vi "Workbench.vi"   [LabVIEW 2024]
uses:
  SDL3/Video/WindowFlags--ring.ctl
  SDL3/Pixels/PixelFormat--enum.ctl
  SDL3/Render/TextureAccess-enum.ctl
  SDL3/Init/InitFlags--ring.ctl
  SDL3/Events/MouseMotionEvent--cluster.ctl
  SDL3/Video/WindowID--integer.ctl
  SDL3/Mouse/MouseID--integer.ctl
  SDL3/Mouse/MouseButtonFlags--ring.ctl
  SDL3/Video/GLAttr--enum.ctl
  SDL3/Render/Vertex--cluster.ctl
  SDL3/Rect/FPoint--cluster.ctl
  SDL3/Pixels/FColor--cluster.ctl
  SDL3/Error/GetError-UiThread.vi
  SDL3/Pixels/PixelFormatEnumToU32.vi
  <vilib>/Utility/error.llb/Error Cluster From Error Code.vi
  SDL3/Init/Init.lvlib
  SDL3/Video/Video.lvlib
  SDL3/Render/Render.lvlib
  SDL3/Pixels/Pixels.lvlib
  SDL3/Timer/Timer.lvlib
  SDL3/Events/Events.lvlib
  SDL3/Mouse/Mouse.lvlib
  SDL3/Rect/Rect.lvlib
  SDL3/Hints/Hints.lvlib
types:
  T1 = typedef "SDL3.lvlib/Video.lvlib/GLAttr--enum.ctl" = enum32{"SDL_GL_RED_SIZE", "SDL_GL_GREEN_SIZE", "SDL_GL_BLUE_SIZE", "SDL_GL_ALPHA_SIZE", "SDL_GL_BUFFER_SIZE", "SDL_GL_DOUBLEBUFFER", "SDL_GL_DEPTH_SIZE", "SDL_GL_STENCIL_SIZE", "SDL_GL_ACCUM_RED_SIZE", "SDL_GL_ACCUM_GREEN_SIZE", "SDL_GL_ACCUM_BLUE_SIZE", "SDL_GL_ACCUM_ALPHA_SIZE", "SDL_GL_STEREO", "SDL_GL_MULTISAMPLEBUFFERS", "SDL_GL_MULTISAMPLESAMPLES", "SDL_GL_ACCELERATED_VISUAL", "SDL_GL_RETAINED_BACKING", "SDL_GL_CONTEXT_MAJOR_VERSION", "SDL_GL_CONTEXT_MINOR_VERSION", "SDL_GL_CONTEXT_FLAGS", "SDL_GL_CONTEXT_PROFILE_MASK", "SDL_GL_SHARE_WITH_CURRENT_CONTEXT", "SDL_GL_FRAMEBUFFER_SRGB_CAPABLE", "SDL_GL_CONTEXT_RELEASE_BEHAVIOR", "SDL_GL_CONTEXT_RESET_NOTIFICATION", "SDL_GL_CONTEXT_NO_ERROR", "SDL_GL_FLOATBUFFERS", "SDL_GL_EGL_PLATFORM"}
  T2 = enum32{"Invalid", "Standard", "Closed", "Hidden", "Minimized", "Maximized"}
  T3 = typedef "SDL3.lvlib/Events.lvlib/MouseMotionEvent--cluster.ctl" = cluster{"timestamp":u64, "windowID":T4, "which":T5, "state":T6, "x":sgl, "y":sgl, "xrel":sgl, "yrel":sgl}
  T4 = typedef "SDL3.lvlib/Video.lvlib/WindowID--integer.ctl" = u32
  T5 = typedef "SDL3.lvlib/Mouse.lvlib/MouseID--integer.ctl" = u32
  T6 = typedef "SDL3.lvlib/Mouse.lvlib/MouseButtonFlags--ring.ctl" = u32
  T7 = typedef "SDL3.lvlib/Init.lvlib/InitFlags--ring.ctl" = u32
  T8 = typedef "SDL3.lvlib/Render.lvlib/TextureAccess-enum.ctl" = enum32{"SDL_TEXTUREACCESS_STATIC", "SDL_TEXTUREACCESS_STREAMING", "SDL_TEXTUREACCESS_TARGET"}
  T9 = typedef "SDL3.lvlib/Pixels.lvlib/PixelFormat--enum.ctl" = enum32{"SDL_PIXELFORMAT_UNKNOWN", "SDL_PIXELFORMAT_INDEX1LSB", "SDL_PIXELFORMAT_INDEX1MSB", "SDL_PIXELFORMAT_INDEX2LSB", "SDL_PIXELFORMAT_INDEX2MSB", "SDL_PIXELFORMAT_INDEX4LSB", "SDL_PIXELFORMAT_INDEX4MSB", "SDL_PIXELFORMAT_INDEX8", "SDL_PIXELFORMAT_RGB332", "SDL_PIXELFORMAT_XRGB4444", "SDL_PIXELFORMAT_XBGR4444", "SDL_PIXELFORMAT_XRGB1555", "SDL_PIXELFORMAT_XBGR1555", "SDL_PIXELFORMAT_ARGB4444", "SDL_PIXELFORMAT_RGBA4444", "SDL_PIXELFORMAT_ABGR4444", "SDL_PIXELFORMAT_BGRA4444", "SDL_PIXELFORMAT_ARGB1555", "SDL_PIXELFORMAT_RGBA5551", "SDL_PIXELFORMAT_ABGR1555", "SDL_PIXELFORMAT_BGRA5551", "SDL_PIXELFORMAT_RGB565", "SDL_PIXELFORMAT_BGR565", "SDL_PIXELFORMAT_RGB24", "SDL_PIXELFORMAT_BGR24", "SDL_PIXELFORMAT_XRGB8888", "SDL_PIXELFORMAT_RGBX8888", "SDL_PIXELFORMAT_XBGR8888", "SDL_PIXELFORMAT_BGRX8888", "SDL_PIXELFORMAT_ARGB8888", "SDL_PIXELFORMAT_RGBA8888", "SDL_PIXELFORMAT_ABGR8888", "SDL_PIXELFORMAT_BGRA8888", "SDL_PIXELFORMAT_XRGB2101010", "SDL_PIXELFORMAT_XBGR2101010", "SDL_PIXELFORMAT_ARGB2101010", "SDL_PIXELFORMAT_ABGR2101010", "SDL_PIXELFORMAT_RGB48", "SDL_PIXELFORMAT_BGR48", "SDL_PIXELFORMAT_RGBA64", "SDL_PIXELFORMAT_ARGB64", "SDL_PIXELFORMAT_BGRA64", "SDL_PIXELFORMAT_ABGR64", "SDL_PIXELFORMAT_RGB48_FLOAT", "SDL_PIXELFORMAT_BGR48_FLOAT", "SDL_PIXELFORMAT_RGBA64_FLOAT", "SDL_PIXELFORMAT_ARGB64_FLOAT", "SDL_PIXELFORMAT_BGRA64_FLOAT", "SDL_PIXELFORMAT_ABGR64_FLOAT", "SDL_PIXELFORMAT_RGB96_FLOAT", "SDL_PIXELFORMAT_BGR96_FLOAT", "SDL_PIXELFORMAT_RGBA128_FLOAT", "SDL_PIXELFORMAT_ARGB128_FLOAT", "SDL_PIXELFORMAT_BGRA128_FLOAT", "SDL_PIXELFORMAT_ABGR128_FLOAT", "SDL_PIXELFORMAT_YV12", "SDL_PIXELFORMAT_IYUV", "SDL_PIXELFORMAT_YUY2", "SDL_PIXELFORMAT_UYVY", "SDL_PIXELFORMAT_YVYU", "SDL_PIXELFORMAT_NV12", "SDL_PIXELFORMAT_NV21", "SDL_PIXELFORMAT_P010", "SDL_PIXELFORMAT_EXTERNAL_OES"}
  T10 = typedef "SDL3.lvlib/Video.lvlib/WindowFlags--ring.ctl" = u64
  T11 = typedef "SDL3.lvlib/Render.lvlib/Vertex--cluster.ctl" = cluster{"Position":T12, "Color":T13, "TexCoord":T12}
  T12 = typedef "SDL3.lvlib/Rect.lvlib/FPoint--cluster.ctl" = cluster{"x":sgl, "y":sgl}
  T13 = typedef "SDL3.lvlib/Pixels.lvlib/FColor--cluster.ctl" = cluster{"r":sgl, "g":sgl, "b":sgl, "a":sgl}
  T14 = typedef "SDL3.lvlib/Events.lvlib/EventType--enum.ctl" = enum16{"LV_NONE", "LV_UNSUPPORTED", "SDL_EVENT_QUIT", "SDL_EVENT_LOCALE_CHANGED", "SDL_EVENT_SYSTEM_THEME_CHANGED", "SDL_EVENT_DISPLAY_ORIENTATION", "SDL_EVENT_DISPLAY_ADDED", "SDL_EVENT_DISPLAY_REMOVED", "SDL_EVENT_DISPLAY_MOVED", "SDL_EVENT_DISPLAY_DESKTOP_MODE_CHANGED", "SDL_EVENT_DISPLAY_CURRENT_MODE_CHANGED", "SDL_EVENT_DISPLAY_CONTENT_SCALE_CHANGED", "SDL_EVENT_WINDOW_SHOWN", "SDL_EVENT_WINDOW_HIDDEN", "SDL_EVENT_WINDOW_EXPOSED", "SDL_EVENT_WINDOW_MOVED", "SDL_EVENT_WINDOW_RESIZED", "SDL_EVENT_WINDOW_PIXEL_SIZE_CHANGED", "SDL_EVENT_WINDOW_METAL_VIEW_RESIZED", "SDL_EVENT_WINDOW_MINIMIZED", "SDL_EVENT_WINDOW_MAXIMIZED", "SDL_EVENT_WINDOW_RESTORED", "SDL_EVENT_WINDOW_MOUSE_ENTER", "SDL_EVENT_WINDOW_MOUSE_LEAVE", "SDL_EVENT_WINDOW_FOCUS_GAINED", "SDL_EVENT_WINDOW_FOCUS_LOST", "SDL_EVENT_WINDOW_CLOSE_REQUESTED", "SDL_EVENT_WINDOW_HIT_TEST", "SDL_EVENT_WINDOW_ICCPROF_CHANGED", "SDL_EVENT_WINDOW_DISPLAY_CHANGED", "SDL_EVENT_WINDOW_DISPLAY_SCALE_CHANGED", "SDL_EVENT_WINDOW_SAFE_AREA_CHANGED", "SDL_EVENT_WINDOW_OCCLUDED", "SDL_EVENT_WINDOW_ENTER_FULLSCREEN", "SDL_EVENT_WINDOW_LEAVE_FULLSCREEN", "SDL_EVENT_WINDOW_DESTROYED", "SDL_EVENT_WINDOW_HDR_STATE_CHANGED", "SDL_EVENT_KEY_DOWN", "SDL_EVENT_KEY_UP", "SDL_EVENT_TEXT_EDITING", "SDL_EVENT_TEXT_INPUT", "SDL_EVENT_KEYMAP_CHANGED", "SDL_EVENT_KEYBOARD_ADDED", "SDL_EVENT_KEYBOARD_REMOVED", "SDL_EVENT_TEXT_EDITING_CANDIDATES", "SDL_EVENT_MOUSE_MOTION", "SDL_EVENT_MOUSE_BUTTON_DOWN", "SDL_EVENT_MOUSE_BUTTON_UP", "SDL_EVENT_MOUSE_WHEEL", "SDL_EVENT_MOUSE_ADDED", "SDL_EVENT_MOUSE_REMOVED", "SDL_EVENT_JOYSTICK_AXIS_MOTION", "SDL_EVENT_JOYSTICK_BALL_MOTION", "SDL_EVENT_JOYSTICK_HAT_MOTION", "SDL_EVENT_JOYSTICK_BUTTON_DOWN", "SDL_EVENT_JOYSTICK_BUTTON_UP", "SDL_EVENT_JOYSTICK_ADDED", "SDL_EVENT_JOYSTICK_REMOVED", "SDL_EVENT_JOYSTICK_BATTERY_UPDATED", "SDL_EVENT_JOYSTICK_UPDATE_COMPLETE", "SDL_EVENT_GAMEPAD_AXIS_MOTION", "SDL_EVENT_GAMEPAD_BUTTON_DOWN", "SDL_EVENT_GAMEPAD_BUTTON_UP", "SDL_EVENT_GAMEPAD_ADDED", "SDL_EVENT_GAMEPAD_REMOVED", "SDL_EVENT_GAMEPAD_REMAPPED", "SDL_EVENT_GAMEPAD_TOUCHPAD_DOWN", "SDL_EVENT_GAMEPAD_TOUCHPAD_MOTION", "SDL_EVENT_GAMEPAD_TOUCHPAD_UP", "SDL_EVENT_GAMEPAD_SENSOR_UPDATE", "SDL_EVENT_GAMEPAD_UPDATE_COMPLETE", "SDL_EVENT_GAMEPAD_STEAM_HANDLE_UPDATED", "SDL_EVENT_FINGER_DOWN", "SDL_EVENT_FINGER_UP", "SDL_EVENT_FINGER_MOTION", "SDL_EVENT_CLIPBOARD_UPDATE", "SDL_EVENT_DROP_FILE", "SDL_EVENT_DROP_TEXT", "SDL_EVENT_DROP_BEGIN", "SDL_EVENT_DROP_COMPLETE", "SDL_EVENT_DROP_POSITION", "SDL_EVENT_AUDIO_DEVICE_ADDED", "SDL_EVENT_AUDIO_DEVICE_REMOVED", "SDL_EVENT_AUDIO_DEVICE_FORMAT_CHANGED", "SDL_EVENT_SENSOR_UPDATE", "SDL_EVENT_PEN_PROXIMITY_IN", "SDL_EVENT_PEN_PROXIMITY_OUT", "SDL_EVENT_PEN_DOWN", "SDL_EVENT_PEN_UP", "SDL_EVENT_PEN_BUTTON_DOWN", "SDL_EVENT_PEN_BUTTON_UP", "SDL_EVENT_PEN_MOTION", "SDL_EVENT_PEN_AXIS", "SDL_EVENT_CAMERA_DEVICE_ADDED", "SDL_EVENT_CAMERA_DEVICE_REMOVED", "SDL_EVENT_CAMERA_DEVICE_APPROVED", "SDL_EVENT_CAMERA_DEVICE_DENIED", "SDL_EVENT_RENDER_TARGETS_RESET", "SDL_EVENT_RENDER_DEVICE_RESET", "SDL_EVENT_POLL_SENTINEL", "SDL_EVENT_USER"}
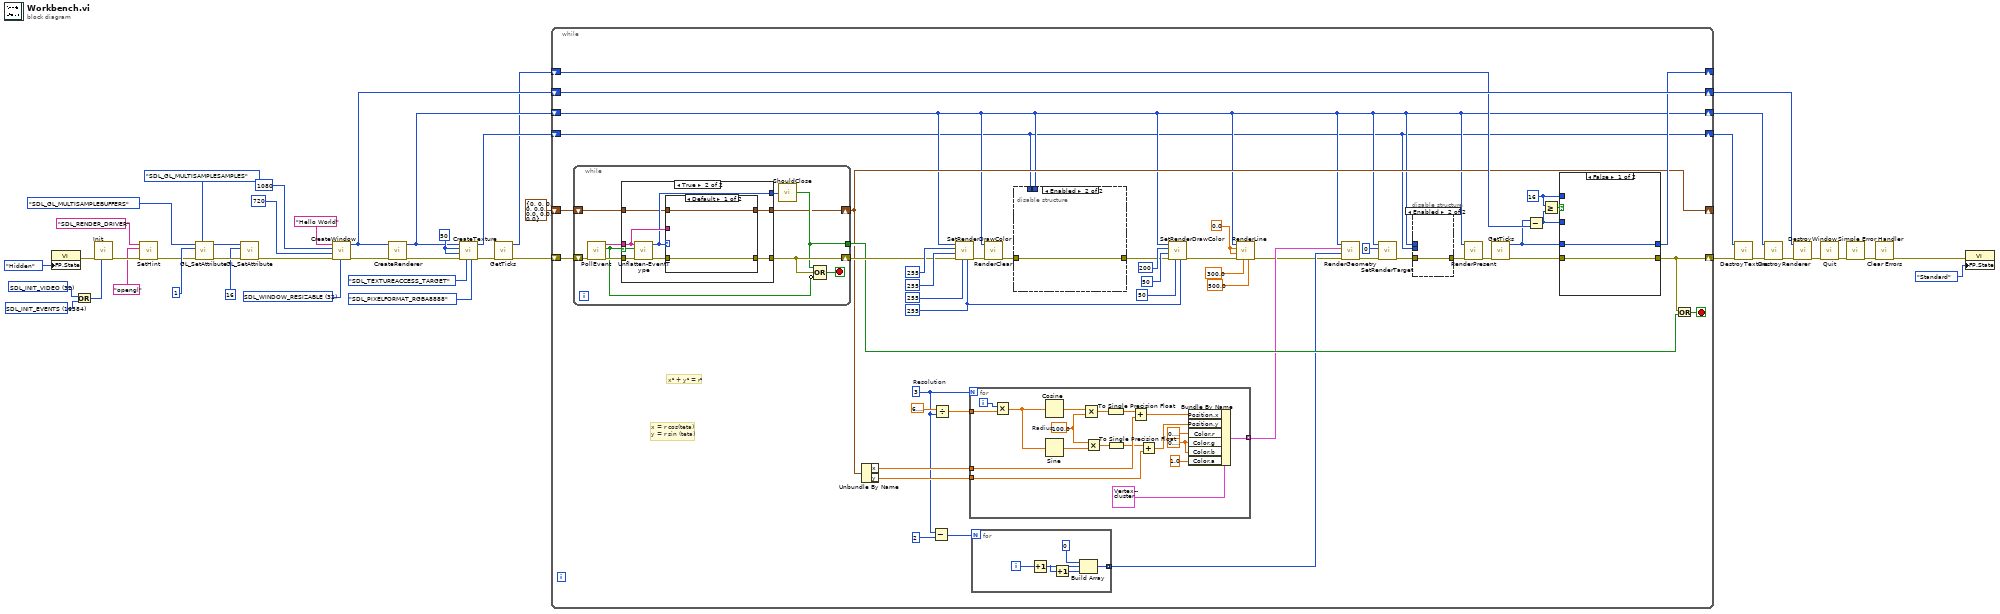
[diagram p0: block diagram]
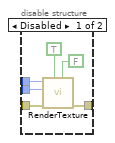
[diagram p2: hidden frame]
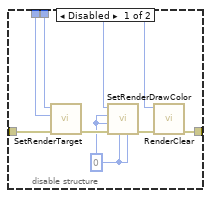
[diagram p3: hidden frame]
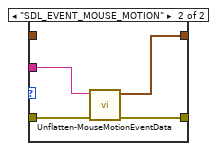
[diagram p5: hidden frame]
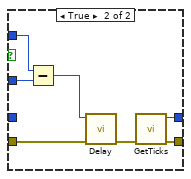
[diagram p6: hidden frame]
diagram:
  w13 = T7 16384 items=["NONE"=0, "SDL_INIT_AUDIO"=16, "SDL_INIT_VIDEO"=32, "SDL_INIT_JOYSTICK"=512, "SDL_INIT_HAPTIC"=4096, "SDL_INIT_GAMEPAD"=8192, "SDL_INIT_EVENTS"=16384, "SDL_INIT_SENSOR"=32768, "SDL_INIT_CAMER"=65536] ("y")
  w18 = T7 32 items=["NONE"=0, "SDL_INIT_AUDIO"=16, "SDL_INIT_VIDEO"=32, "SDL_INIT_JOYSTICK"=512, "SDL_INIT_HAPTIC"=4096, "SDL_INIT_GAMEPAD"=8192, "SDL_INIT_EVENTS"=16384, "SDL_INIT_SENSOR"=32768, "SDL_INIT_CAMER"=65536] ("InitFlags")
  w35 = 50 ("w")
  w40 = T10 32 items=["0"=0, "SDL_WINDOW_FULLSCREEN"=1, "SDL_WINDOW_OPENGL"=2, "SDL_WINDOW_OCCLUDED"=4, "SDL_WINDOW_HIDDEN"=8, "SDL_WINDOW_BORDERLESS"=16, "SDL_WINDOW_RESIZABLE"=32, "SDL_WINDOW_MINIMIZED"=64, "SDL_WINDOW_MAXIMIZED"=128, "SDL_WINDOW_MOUSE_GRABBED"=256, "SDL_WINDOW_INPUT_FOCUS"=512, "SDL_WINDOW_MOUSE_FOCUS"=1024, "SDL_WINDOW_EXTERNAL"=2048, "SDL_WINDOW_MODAL"=4096, "SDL_WINDOW_HIGH_PIXEL_DENSITY"=8192, "SDL_WINDOW_MOUSE_CAPTURE"=16384, "SDL_WINDOW_MOUSE_RELATIVE_MODE"=32768, "SDL_WINDOW_ALWAYS_ON_TOP"=65536, "SDL_WINDOW_UTILITY"=131072, "SDL_WINDOW_TOOLTIP"=262144, "SDL_WINDOW_POPUP_MENU"=524288, "SDL_WINDOW_KEYBOARD_GRABBED"=1048576, "SDL_WINDOW_VULKAN"=268435456, "SDL_WINDOW_METAL"=536870912, "SDL_WINDOW_TRANSPARENT"=1073741824, "SDL_WINDOW_NOT_FOCUSABLE"=2147483648] ("flags (0)")
  n1 = property class="VI"("FP.State"=T2."Hidden" ("Front Panel Window:State")) -> (error out=w23:errorcluster)  [unwired: 2 in, 1 out]
  n2 = Or(x=w18, y=w13) -> (x .or. y?=w14:T7)
  n3 = call "Init.vi"("InitFlags"=w14, "No Error"=w23) -> ("error out"=w10:errorcluster)  [unwired: 9 in]
  n4 = call "SetHint.vi"("No Error"=w10, "Value"="opengl", "Hint Name"="SDL_RENDER_DRIVER") -> ("error out"=w3:errorcluster)  [unwired: 8 in]
  n5 = call "GL_SetAttribute.vi"("No Error"=w3, "Value"=1, "GL Attribute"=GLAttr--enum."SDL_GL_MULTISAMPLEBUFFERS") -> ("Error Out"=w8:errorcluster)  [unwired: 8 in]
  n6 = call "GL_SetAttribute.vi"("No Error"=w8, "Value"=16, "GL Attribute"=GLAttr--enum."SDL_GL_MULTISAMPLESAMPLES") -> ("Error Out"=w9:errorcluster)  [unwired: 8 in]
  n7 = call "CreateWindow.vi"("Flags (0)"=w40, "No Error"=w9, "H"=720 ("h"), "W"=1080 ("w"), "Title"="Hello World" ("title")) -> ("Error Out"=w39:errorcluster, "Window [SDL_Window *]"=w31:i64)  [unwired: 5 in]
  n8 = call "CreateRenderer.vi"("No Error"=w39, "Window [SDL_Window *]"=w31) -> ("Error Out"=w36:errorcluster, "Renderer [SDL_Renderer *]"=w30:i64)  [unwired: 8 in]
  n9 = call "CreateTexture.vi"("Pixel Format"=PixelFormat--enum."SDL_PIXELFORMAT_RGBA8888" ("pixel_format"), "Texture Access"=TextureAccess-enum."SDL_TEXTUREACCESS_TARGET" ("texture_access"), "No Error"=w36, "H"=w35, "W"=w35, "Renderer [SDL_Renderer *]"=w30) -> ("error out"=w17:errorcluster, "Texture [SDL_Texture *]"=w29:i64)  [unwired: 4 in]
  n10 = call "GetTicks.vi"("No Error"=w17) -> ("error out"=w16:errorcluster, "Ticks [ms]"=w15:u64)  [unwired: 9 in]
  n11 = while {
    shift-right: [w43] -> w26
    shift-left: w29 -> [w43]
    shift-right: [w47] -> w27
    shift-left: w30 -> [w47]
    shift-right: [w88] -> w28
    shift-left: w31 -> [w88]
    shift-right: [w59] -> w38
    shift-left: w16 -> [w67]
    shift-right: [w75] -> _
    shift-left: w15 -> [w72]
    shift-right: [w58] -> _
    shift-left: T3 {"timestamp"=0, "windowID"=0, "which"=0, "state"=0, "x"=0.0, "y"=0.0, "xrel"=0.0, "yrel"=0.0} ("MouseMotionEvent") -> [w66]
    stop <- w60 stop-if-true
    w46 = sgl 0.0 ("X1")
    w52 = 3  # Resolution
    w71 = u64 16
    w63 = u8 255 ("a")
    # "x = r cos(teta)\ny = r sin (teta)"
    # "x² + y² = r²"
    n12 = while {
      shift-right: [w132] -> w65
      shift-left: w67 -> [w137]
      tunnel: [w130] -> w61
      shift-right: [w129] -> w58
      shift-left: w66 -> [w128]
      stop <- w136 stop-if-true
      n13 = call "PollEvent.vi"("No Error"=w137) -> ("error out"=w135:errorcluster, "Event Occured?"=w133:bool, "Event Binary Data"=w134:string)  [unwired: 8 in]
      n14 = case shown="True" w133 {
        tunnel: w135 -> [w139 w146]
        tunnel: w134 -> [_ w145]
        tunnel: [w139 w142] -> w132
        tunnel: [_ w144] -> w131
        tunnel: [w138 w141] -> w129
        tunnel: w128 -> [w138 w140]
        frame False {
        }
        frame True {
          n15 = call "Unflatten-EventType.vi"("error in (no error)"=w146, "Event Binary Data In"=w145) -> ("error out"=w143:errorcluster, "EventType"=w144:T14)  [unwired: 8 in]
          n16 = case shown="Default" w144 {
            tunnel: w145 -> [_ w151]
            tunnel: w143 -> [w148 w152]
            tunnel: [w148 w150] -> w142
            tunnel: [w147 w149] -> w141
            tunnel: w140 -> [w147 _]
            frame Default {
            }
            frame "SDL_EVENT_MOUSE_MOTION" {
              n17 = call "Unflatten-MouseMotionEventData.vi"("error in (no error)"=w152, "Event Binary Data"=w151) -> ("error out"=w150:errorcluster, "MouseMotionEvent"=w149:T3)  [unwired: 8 in]
            }
          }
        }
      }
      n18 = call "ShouldClose.vi"("EventType"=w131) -> ("Close?"=w130:bool)
      n19 = Compound Arithmetic op=OR(w130, w132, invert w133) -> (w136:bool)
    }
    n20 = Unbundle By Name(w58) -> ("x"=w57:sgl, "y"=w56:sgl)
    n21 = Subtract(x=w52, y=2) -> (x-y=w51:i32)
    n22 = Divide(x=6.283185307179586, y=w52) -> (x/y=w53:dbl)
    n23 = call "SetRenderDrawColor.vi"("A"=w63, "B"=u8 255 ("b"), "No Error"=w65, "G"=u8 255 ("g"), "R"=u8 255 ("r"), "Renderer [SDL_Renderer *]"=w47) -> ("error out"=w85:errorcluster)  [unwired: 5 in]
    n24 = for {
      N: w52 -> [_]
      tunnel: w53 -> [w111]
      tunnel: w57 -> [w105]
      tunnel: w56 -> [w103]
      tunnel: [w94] -> w55 mode=indexing
      i -> [w112]
      w96 = sgl 0.1 ("Color.g")
      w107 = 100.0  # Radius
      n25 = Multiply(x=w112, y=w111) -> (x*y=w110:dbl)
      n26 = Cosine(x=w110) -> (cos(x)=w109:dbl)
      n27 = Sine(x=w110) -> (sin(x)=w108:dbl)
      n28 = Multiply(x=w109, y=w107) -> (x*y=w106:dbl)
      n29 = Multiply(x=w107, y=w108) -> (x*y=w104:dbl)
      n30 = To Single Precision Float(number=w106) -> (single precision float=w99:sgl)
      n31 = To Single Precision Float(number=w104) -> (single precision float=w98:sgl)
      n32 = Add(x=w99, y=w105) -> (x+y=w101:sgl)
      n33 = Add(x=w98, y=w103) -> (x+y=w100:sgl)
      n34 = Bundle By Name(cluster=T11 {"Position"={"x"=0.0, "y"=0.0}, "Color"={"r"=0.0, "g"=0.0, "b"=0.0, "a"=0.0}, "TexCoord"={"x"=0.0, "y"=0.0}} ("Vertex"), "Position.x"=w101, "Position.y"=w100, "Color.r"=sgl 0.8, "Color.g"=w96, "Color.b"=w96, "Color.a"=sgl 1.0) -> (w94:T11)
    }
    n35 = for {
      N: w51 -> [_]
      tunnel: [w89] -> w49 mode=concatenating
      i -> [w93]
      n36 = Increment(x=w93) -> (x+1=w92:i32)
      n37 = Increment(x=w92) -> (x+1=w91:i32)
      n38 = Build Array(0 ("element"), w92, w91) -> (w89:i32[])
    }
    n39 = call "RenderClear.vi"("No Error"=w85, "Renderer [SDL_Renderer *]"=w47) -> ("error out"=w64:errorcluster)  [unwired: 9 in]
    n40 = disable-structure shown="Enabled" {
      disable-tunnel: w64 -> [w126 w127]
      disable-tunnel: w43 -> [w125 _]
      disable-tunnel: [w122 w127] -> w62
      disable-tunnel: w47 -> [w121 _]
      frame Disabled {
        w120 = u8 0 ("r")
        n41 = call "SetRenderTarget.vi"("No Error"=w126, "Texture [SDL_Texture *]"=w125, "Renderer [SDL_Renderer *]"=w121) -> ("error out"=w124:errorcluster)  [unwired: 8 in]
        n42 = call "SetRenderDrawColor.vi"("A"=w120, "B"=w120, "No Error"=w124, "G"=w120, "R"=w120, "Renderer [SDL_Renderer *]"=w121) -> ("error out"=w123:errorcluster)  [unwired: 5 in]
        n43 = call "RenderClear.vi"("No Error"=w123, "Renderer [SDL_Renderer *]"=w121) -> ("error out"=w122:errorcluster)  [unwired: 9 in]
      }
      frame Enabled {
      }
    }
    n44 = call "SetRenderDrawColor.vi"("A"=w63, "B"=u8 50 ("b"), "No Error"=w62, "G"=u8 50 ("g"), "R"=u8 200 ("r"), "Renderer [SDL_Renderer *]"=w47) -> ("error out"=w80:errorcluster)  [unwired: 5 in]
    n45 = call "RenderLine.vi"("Y2"=sgl 500.0 ("X2"), "X2"=sgl 300.0, "No Error"=w80, "Y1"=w46, "X1"=w46, "Renderer [SDL_Renderer *]"=w47) -> ("error out"=w48:errorcluster)  [unwired: 5 in]
    n46 = call "RenderGeometry.vi"("No Error"=w48, "Indices (Empty)"=w49, "Vertices"=w55, "Renderer [SDL_Renderer *]"=w47) -> ("error out"=w76:errorcluster)  [unwired: 7 in]
    n47 = call "SetRenderTarget.vi"("No Error"=w76, "Texture [SDL_Texture *]"=i64 0 ("texture [SDL_Texture *]"), "Renderer [SDL_Renderer *]"=w47) -> ("error out"=w86:errorcluster)  [unwired: 8 in]
    n48 = disable-structure shown="Enabled" {
      disable-tunnel: [w118 w119] -> w87
      disable-tunnel: w86 -> [w117 w119]
      disable-tunnel: w43 -> [w114 _]
      disable-tunnel: w47 -> [w113 _]
      frame Disabled {
        n49 = call "RenderTexture.vi"("Entire Rendering Target (F)"=FALSE, "Entire Texture (F)"=TRUE, "No Error"=w117, "Texture [SDL_Texture *]"=w114, "Renderer [SDL_Renderer *]"=w113) -> ("error out"=w118:errorcluster)  [unwired: 6 in]
      }
      frame Enabled {
      }
    }
    n50 = call "RenderPresent.vi"("No Error"=w87, "Renderer [SDL_Renderer *]"=w47) -> ("error out"=w74:errorcluster)  [unwired: 9 in]
    n51 = call "GetTicks.vi"("No Error"=w74) -> ("error out"=w73:errorcluster, "Ticks [ms]"=w68:u64)  [unwired: 9 in]
    n52 = Subtract(x=w68, y=w72) -> (x-y=w70:u64)
    n53 = Greater Or Equal?(x=w71, y=w70) -> (x >= y?=w69:bool)
    n54 = case shown="False" w69 {
      tunnel: [w153 w161] -> w59
      tunnel: [w154 w160] -> w75
      tunnel: w73 -> [w153 w159]
      tunnel: w71 -> [_ w158]
      tunnel: w70 -> [_ w157]
      tunnel: w68 -> [w154 _]
      frame False {
      }
      frame True {
        n55 = Subtract(x=w158, y=w157) -> (x-y=w155:u64)
        n56 = call "Delay.vi"("No Error"=w159, "ms"=w155) -> ("error out"=w156:errorcluster)  [unwired: 9 in]
        n57 = call "GetTicks.vi"("No Error"=w156) -> ("error out"=w161:errorcluster, "Ticks [ms]"=w160:u64)  [unwired: 9 in]
      }
    }
    n58 = Or(x=w59, y=w61) -> (x .or. y?=w60:bool)
  }
  n59 = call "DestroyTexture.vi"("No Error"=w38, "Texture [SDL_Texture *]"=w26) -> ("error out"=w32:errorcluster)  [unwired: 9 in]
  n60 = call "DestroyRenderer.vi"("No Error"=w32, "Rrenderer [SDL_Renderer *]"=w27) -> ("error out"=w37:errorcluster)  [unwired: 9 in]
  n61 = call "DestroyWindow.vi"("No Error"=w37, "Window [SDL_Window*]"=w28) -> ("Error Out"=w42:errorcluster)  [unwired: 9 in]
  n62 = call "Quit.vi"("No Error"=w42) -> ("error out"=w21:errorcluster)  [unwired: 10 in]
  n63 = call <vilib>:"Simple Error Handler.vi"("error in (no error)"=w21) -> ("error out"=w20:errorcluster)  [unwired: 4 in, 4 out]
  n64 = call <vilib>:"Clear Errors.vi"("error in (no error)"=w20) -> ("error out"=w19:errorcluster)  [unwired: 5 in, 1 out]
  n65 = property class="VI"(error in=w19, "FP.State"=T2."Standard" ("Front Panel Window:State")) -> ()  [unwired: 1 in, 2 out]
